vi "SSC DCPower Configure Aperture Time with Abort and Initiate.vi"(0 "DCPower SSC in":T1[](array[typedef]), 5 "Aperture Times":dbl format="%#_6p", 7 "Aperture Time Units":T2=1028 caption="aperture time units" items=["Seconds"=1028, "Powerline Cycles"=1029], 11 "error in":errorcluster) -> (4 "DCPower SSC out":T1[](array[typedef]), 15 "error out":errorcluster)   [LabVIEW 2019]
doc: "This VI aborts, configures measurement aperture time, and initializes the sessions."
uses:
  <instrlib>/niDCPower/nidcpower.llb/niDCPower Aperture Time Units.ctl
  SSC DCPower.ctl
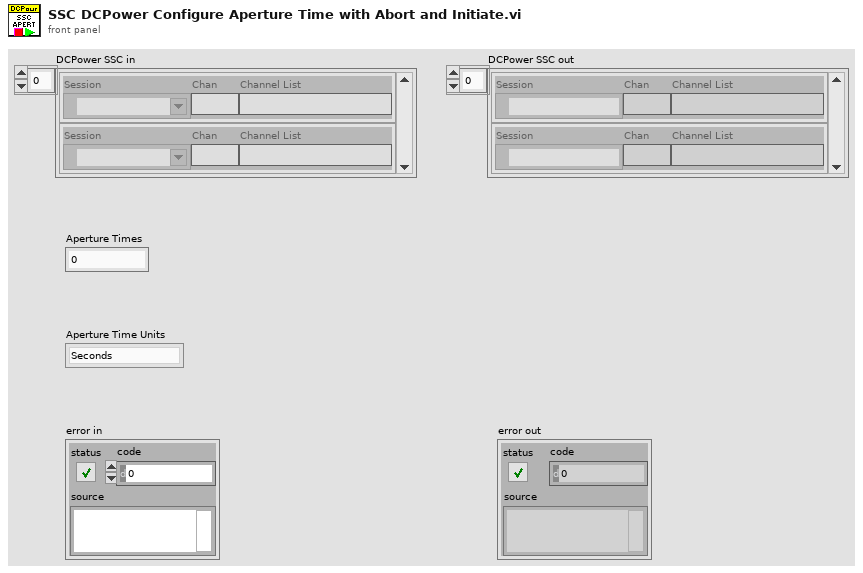
[diagram p1: front panel]
types:
  T1 = typedef "SSC DCPower.ctl" = cluster{"Session":refnum<k15>, "Chan":string, "Channel List":string}
  T2 = typedef "niDCPower Aperture Time Units.ctl" = i32
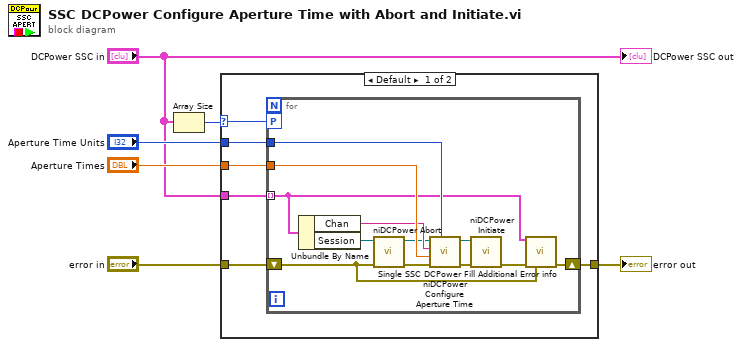
[diagram p0: block diagram]
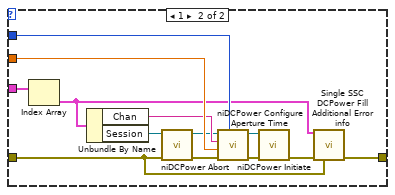
[diagram p2: hidden frame]
diagram:
  n1 = Array Size(array="DCPower SSC in") -> (size(s)=w2:i32)
  n2 = case shown="Default" w2 {
    selector: w2 -> [w8 _]
    tunnel: "error in" -> [w12 w37]
    tunnel: [w11 w36] -> w5
    tunnel: "Aperture Times" -> [w10 w35]
    tunnel: "Aperture Time Units" -> [w9 w34]
    tunnel: "DCPower SSC in" -> [w7 w33]
    frame Default {
      n3 = for {
        tunnel: w7 -> [w14] mode=indexing
        workers-P: w8 -> [_]
        tunnel: w9 -> [w23]
        tunnel: w10 -> [w24]
        shift-right: [w15] -> w11
        shift-left: w12 -> [w13]
        n4 = Unbundle By Name(w14) -> ("Chan"=w21:string, "Session"=w18:refnum<k15>)
        n5 = call <instrlib>:"niDCPower Abort.vi"("error in (no error)"=w13, "instrument handle"=w18) -> ("error out"=w19:errorcluster, "instrument handle out"=w17:refnum<k15>)  [unwired: 8 in]
        n6 = call <instrlib>:"niDCPower Configure Aperture Time.vi"("aperture time units"=w23, "error in (no error)"=w19, "aperture time"=w24, "channel name"=w21, "instrument handle"=w17) -> ("error out"=w20:errorcluster, "instrument handle out"=w16:refnum<k15>)  [unwired: 5 in]
        n7 = call <instrlib>:"niDCPower Initiate.vi"("error in (no error)"=w20, "instrument handle"=w16) -> ("error out"=w22:errorcluster)  [unwired: 8 in, 1 out]
        n8 = call "Single SSC DCPower Fill Additional Error info.vi"("DCPower SSC in"=w14, "error in"=w22, "previous error in"=w13) -> ("error out"=w15:errorcluster)  [unwired: 12 in]
      }
    }
    frame 1 {
      n9 = Index Array(array=w33) -> (element=w25:T1)  [unwired: 1 in]
      n10 = Unbundle By Name(w25) -> ("Chan"=w31:string, "Session"=w28:refnum<k15>)
      n11 = call <instrlib>:"niDCPower Abort.vi"("error in (no error)"=w37, "instrument handle"=w28) -> ("error out"=w29:errorcluster, "instrument handle out"=w27:refnum<k15>)  [unwired: 8 in]
      n12 = call <instrlib>:"niDCPower Configure Aperture Time.vi"("aperture time units"=w34, "error in (no error)"=w29, "aperture time"=w35, "channel name"=w31, "instrument handle"=w27) -> ("error out"=w30:errorcluster, "instrument handle out"=w26:refnum<k15>)  [unwired: 5 in]
      n13 = call <instrlib>:"niDCPower Initiate.vi"("error in (no error)"=w30, "instrument handle"=w26) -> ("error out"=w32:errorcluster)  [unwired: 8 in, 1 out]
      n14 = call "Single SSC DCPower Fill Additional Error info.vi"("DCPower SSC in"=w25, "error in"=w32, "previous error in"=w37) -> ("error out"=w36:errorcluster)  [unwired: 12 in]
    }
  }
  "error out" <- w5
  "DCPower SSC out" <- "DCPower SSC in"
